vi "GlobalRECORD22.vi"() -> ()   [LabVIEW 2021]
panel:
  out "record":bool
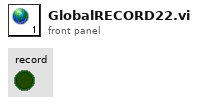
[diagram p1: front panel]
diagram:
